vi "SupportedMetricsFor60sBlock.vi"() -> (3 "Supported Metrics":string[](array[string]))   [LabVIEW 2016, in "McsaAnalysisFunctions.lvlib"]
uses:
  <vilib>/addons/InsightCM/Utilities/Analysis/MCSA/McsaAnalysisFunctions.lvlib
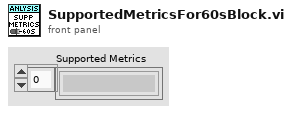
[diagram p1: front panel]
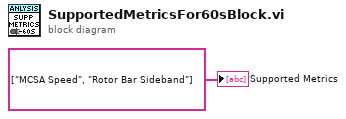
[diagram p0: block diagram]
diagram:
  "Supported Metrics" <- string[] ["MCSA Speed", "Rotor Bar Sideband"] ("value")
